vi "enqueueAllFront.vi"(1 "Waypoint Queue":refnum<queue>, 2 "timeout in ms (-1)":i32, 3 "Waypoint Array":refnum<class "Waypoint.lvclass">[](array[class])) -> (0 "Waypoint Queue Out":refnum<queue>)   [LabVIEW 2013]
doc: "Enqueues an array of waypoints to the front of the queue\n\nJoe Sutker\n4 Dec 2014"
uses:
  Logic/Classes/Waypoint/Waypoint.lvclass
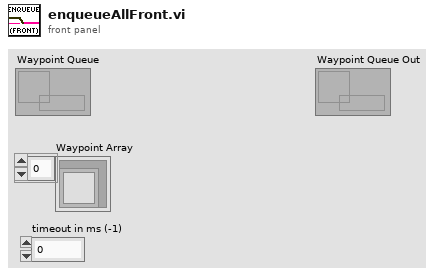
[diagram p1: front panel]
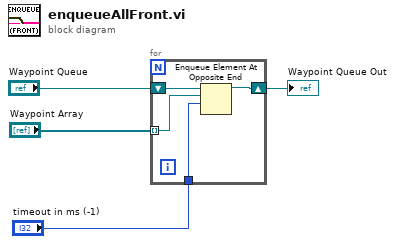
[diagram p0: block diagram]
diagram:
  n1 = for {
    shift-right: [w7] -> w3
    shift-left: "Waypoint Queue" -> [w8]
    tunnel: "Waypoint Array" -> [w6] mode=indexing
    tunnel: "timeout in ms (-1)" -> [w5]
    n2 = Enqueue Element At Opposite End(queue=w8, element=w6, timeout in ms (-1)=w5) -> (queue out=w7:refnum<queue>)  [unwired: 1 in, 2 out]
  }
  "Waypoint Queue Out" <- w3
